vi "IRSensorConvSubVI.vi"(11 "Infrared Sensor Reading":fxp<+/-,25,5>) -> (3 "Sensor Data":dbl)   [LabVIEW 2013]
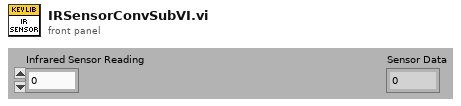
[diagram p1: front panel]
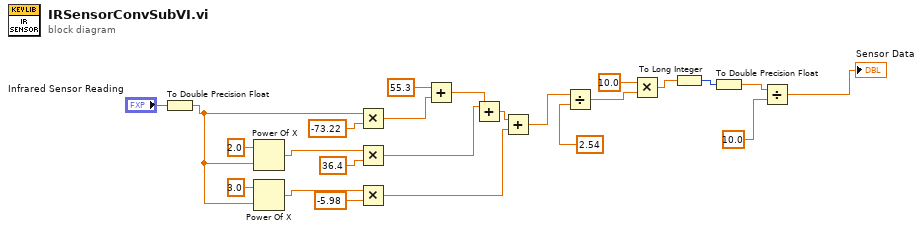
[diagram p0: block diagram]
diagram:
  n1 = To Double Precision Float(number="Infrared Sensor Reading") -> (double precision float=w21:dbl)
  n2 = Power Of X(1:w21, 2:2.0 ("y")) -> (0:w20:dbl)
  n3 = Power Of X(1:w21, 2:3.0 ("y")) -> (0:w19:dbl)
  n4 = Multiply(x=w21, y=-73.22) -> (x*y=w14:dbl)
  n5 = Multiply(x=w20, y=36.4) -> (x*y=w12:dbl)
  n6 = Multiply(x=w19, y=-5.98) -> (x*y=w10:dbl)
  n7 = Add(x=55.3, y=w14) -> (x+y=w13:dbl)
  n8 = Add(x=w12, y=w13) -> (x+y=w11:dbl)
  n9 = Add(x=w11, y=w10) -> (x+y=w8:dbl)
  n10 = Divide(x=w8, y=2.54) -> (x/y=w7:dbl)
  n11 = Multiply(x=10.0, y=w7) -> (x*y=w5:dbl)
  n12 = To Long Integer(number=w5) -> (32bit integer=w4:i32)
  n13 = To Double Precision Float(number=w4) -> (double precision float=w3:dbl)
  n14 = Divide(x=w3, y=10.0) -> (x/y=→"Sensor Data":dbl)
